vi "Write Iterations.vi"(8 "error in (no error)":errorcluster, 10 "Iterations":u16, 11 "Termination Criteria in":refnum<class "Termination Criteria.lvclass">) -> (0 "error out":errorcluster, 3 "Termination Criteria out":refnum<class "Termination Criteria.lvclass">)   [LabVIEW 2020, in "g_ar_toolkit.common.lvlib" / "Termination Criteria.lvclass"]
uses:
  Termination Criteria.lvclass
  Termination Criteria.lvclass/Termination Criteria.ctl
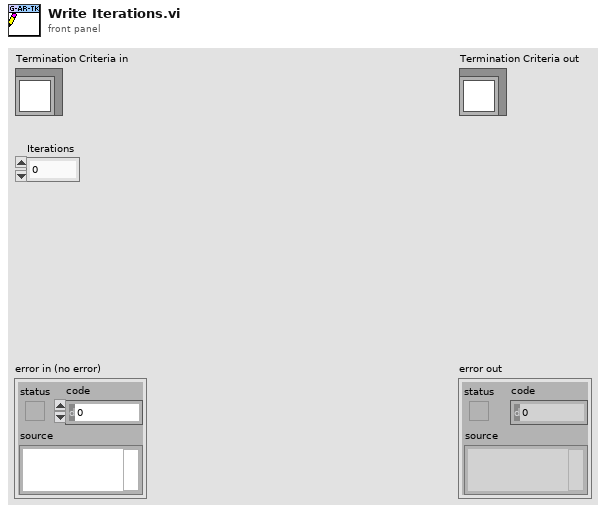
[diagram p1: front panel]
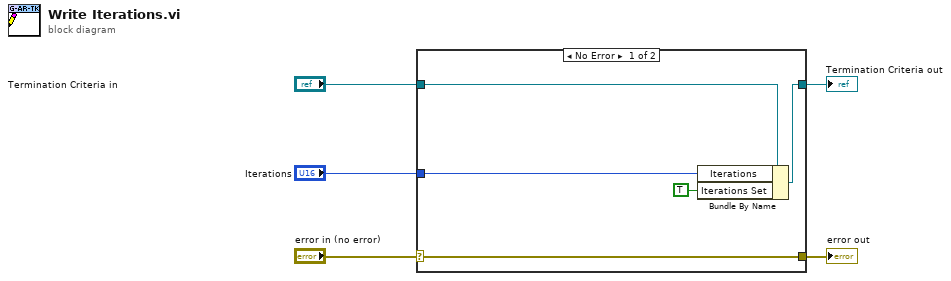
[diagram p0: block diagram]
diagram:
  n1 = case shown="No Error" "error in (no error)" {
    selector: "error in (no error)" -> [w10 w11]
    tunnel: [w10 w11] -> w4
    tunnel: [w8 w12] -> w2
    tunnel: "Termination Criteria in" -> [w9 w12]
    tunnel: "Iterations" -> [w7 _]
    frame No Error {
      n2 = Bundle By Name(cluster=w9, "Iterations"=w7, "Iterations Set"=TRUE) -> (w8:refnum<class "Termination Criteria.lvclass">)
    }
    frame Error {
    }
  }
  "error out" <- w4
  "Termination Criteria out" <- w2
